vi "lapdata_new.vi"(6 "Reset":bool, 7 "Laptrigger":bool, 8 "InverterTemps":dbl[](array[numeric]), 9 "MotorTemps":dbl[](array[numeric]), 10 "Current":dbl, 11 "Hv Data":dbl[](array[numeric])) -> (0 "Inverter Temp":cluster{i32[], dbl[]}[](graph), 1 "Motor Temp":cluster{i32[], dbl[]}[](graph), 2 "HV Temps":dbl[](array[numeric]), 3 "Lap                    Laptime                        SoC                 Current Avg |                             Motor Temperatures                          |                               Inverter Temperatures":T1(array[cluster]) {"Laptime" format="%<%M:%S%2u>T"})   [LabVIEW 2017]
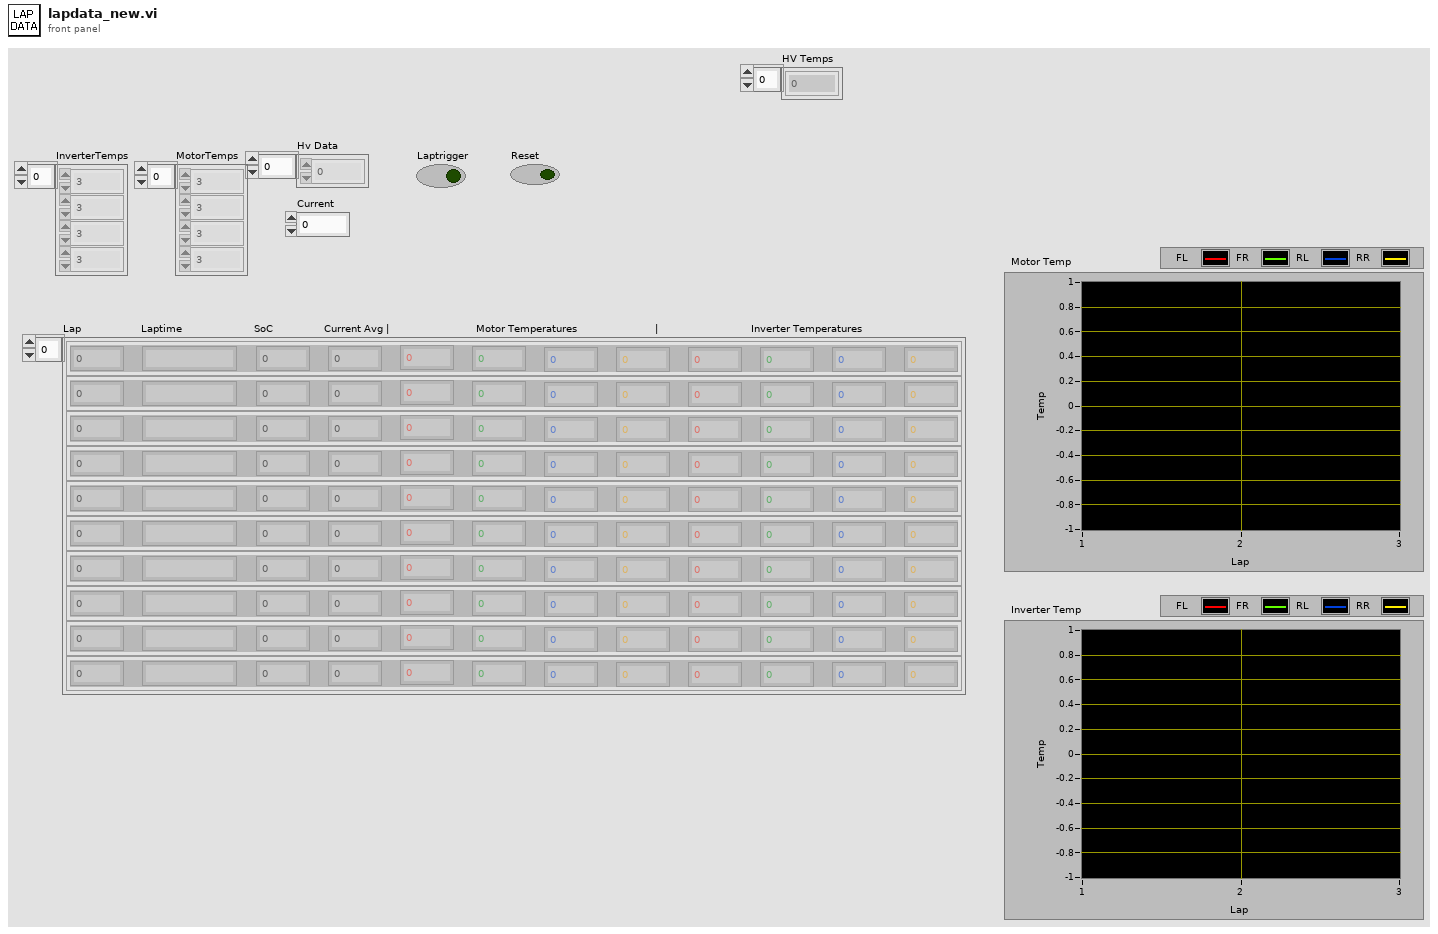
[diagram p1: front panel]
types:
  T1 = cluster{"SoC":i32, "MotorTemp_FL":dbl, "MotorTemp_FR":dbl, "MotorTemp_RL":dbl, "MotorTemp_RR":dbl, "InverterTemp_FL":dbl, "InverterTemp_FR":dbl, "InverterTemp_RL":dbl, "InverterTemp_RR":dbl, "Laptime":timestamp, "Lap":i32, "Curr Abs Avg":dbl}[]
  T2 = cluster{"SoC":i32, "MotorTemp_FL":dbl, "MotorTemp_FR":dbl, "MotorTemp_RL":dbl, "MotorTemp_RR":dbl, "InverterTemp_FL":dbl, "InverterTemp_FR":dbl, "InverterTemp_RL":dbl, "InverterTemp_RR":dbl, "Laptime":timestamp, "Lap":i32, "Current Abs Avg":dbl, "HV Temp":dbl}[]
  T3 = cluster{"SoC":i32, "MotorTemp_FL":dbl, "MotorTemp_FR":dbl, "MotorTemp_RL":dbl, "MotorTemp_RR":dbl, "InverterTemp_FL":dbl, "InverterTemp_FR":dbl, "InverterTemp_RL":dbl, "InverterTemp_RR":dbl, "Laptime":timestamp, "Lap":i32, "Current Abs Avg":dbl, "HV Temp":dbl}
  T4 = cluster{"SoC":i32, "MotorTemp_FL":dbl, "MotorTemp_FR":dbl, "MotorTemp_RL":dbl, "MotorTemp_RR":dbl, "InverterTemp_FL":dbl, "InverterTemp_FR":dbl, "InverterTemp_RL":dbl, "InverterTemp_RR":dbl, "Laptime":timestamp, "Lap":i32, "Current Abs Avg":dbl}
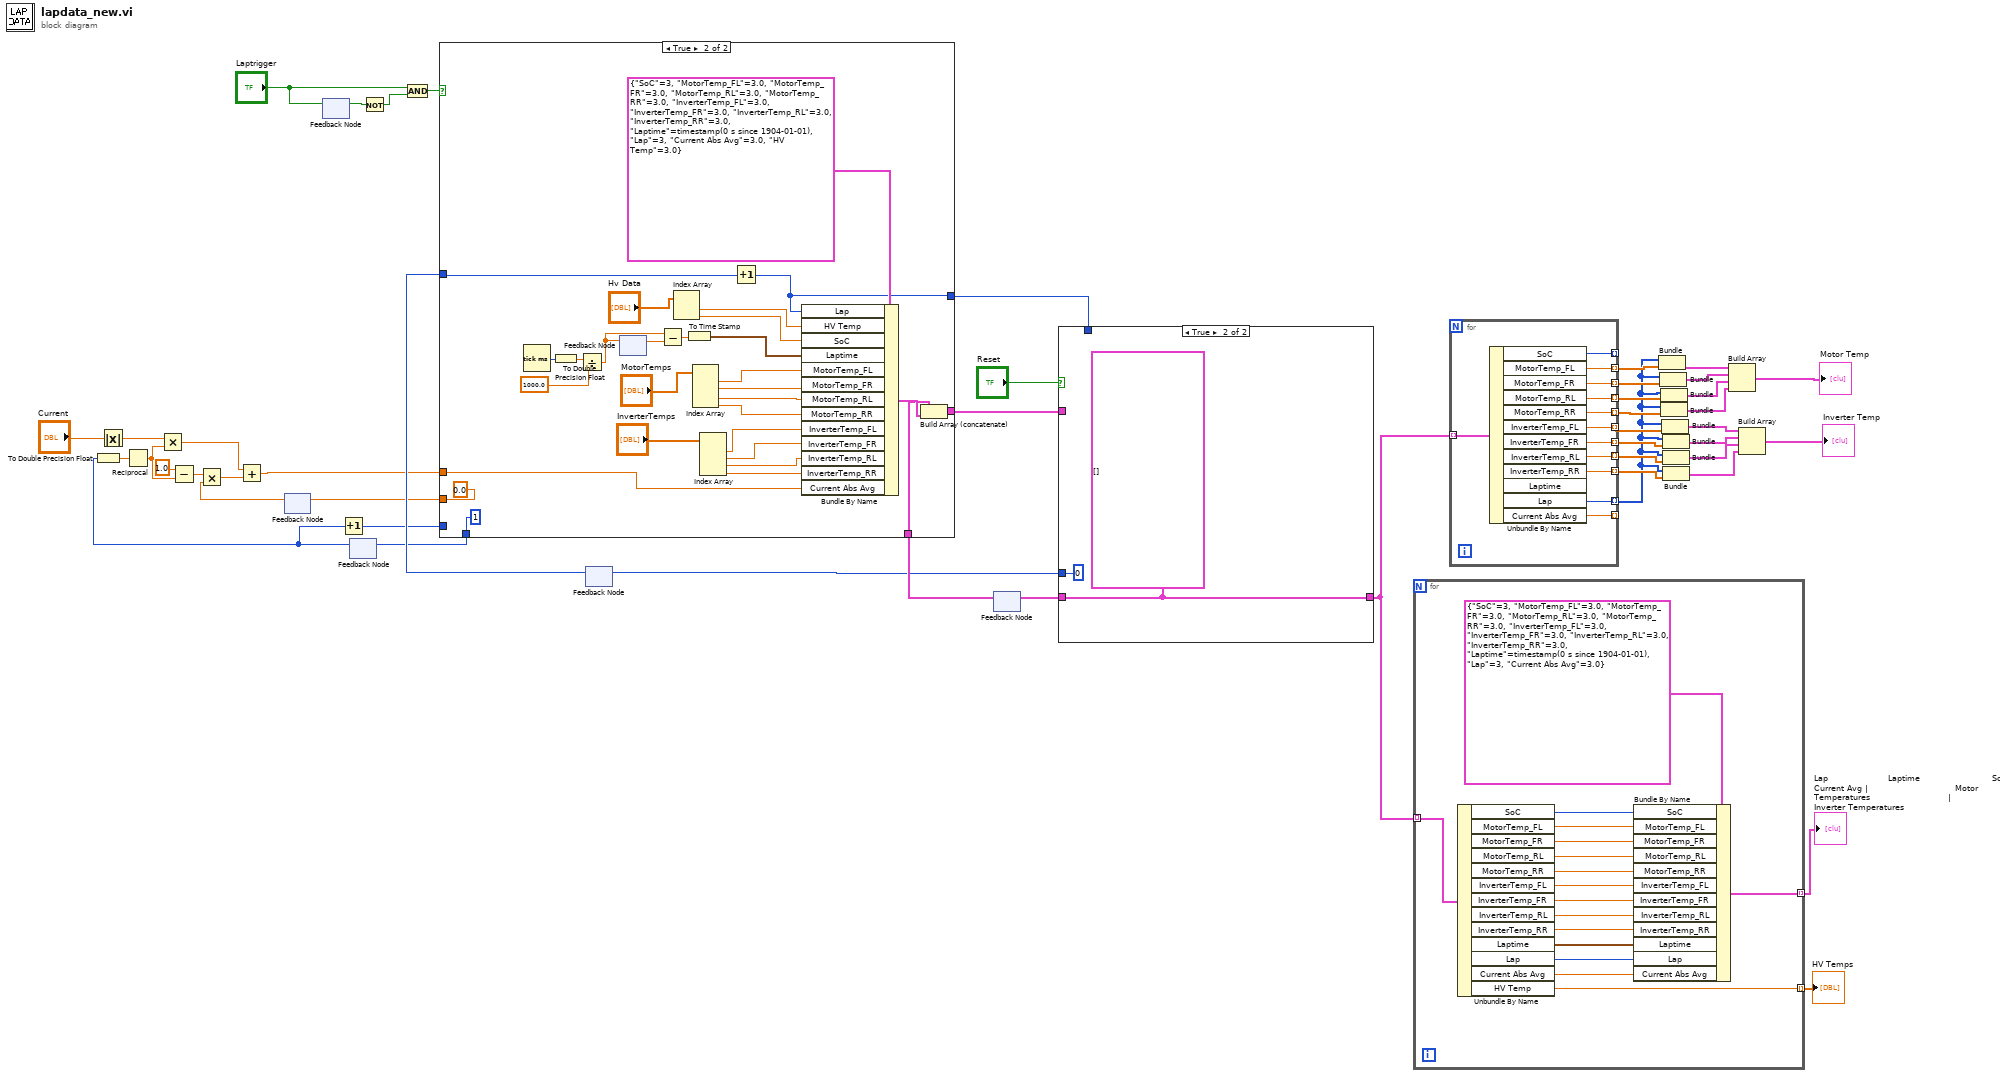
[diagram p0: block diagram]
diagram:
  n1 = Absolute Value(x="Current") -> (abs(x)=w28:dbl)
  n2 = feedback #1() -> (w32:dbl)  [unwired: 1 in]
  n3 = feedback #2() -> (w46:bool)  [unwired: 1 in]
  n4 = feedback-in #2("Laptrigger") -> ()
  n5 = feedback #3() -> (w35:i32)  [unwired: 1 in]
  n6 = To Double Precision Float(number=w35) -> (double precision float=w36:dbl)
  n7 = Reciprocal(x=w36) -> (1/x=w30:dbl)
  n8 = Multiply(x=w28, y=w30) -> (x*y=w34:dbl)
  n9 = Subtract(x=1.0, y=w30) -> (x-y=w31:dbl)
  n10 = Multiply(x=w31, y=w32) -> (x*y=w33:dbl)
  n11 = Add(x=w34, y=w33) -> (x+y=w24:dbl)
  n12 = Increment(x=w35) -> (x+1=w26:i32)
  n13 = Not(x=w46) -> (.not. x?=w45:bool)
  n14 = And(x="Laptrigger", y=w45) -> (x .and. y?=w43:bool)
  n15 = feedback #4() -> (w37:i32)  [unwired: 1 in]
  n16 = feedback #5() -> (w47:T2)  [unwired: 1 in]
  n17 = case shown="True" w43 {
    tunnel: w47 -> [w51 w60]
    tunnel: [w51 w79] -> w41
    tunnel: [w50 w53] -> w39
    tunnel: w37 -> [w50 w59]
    tunnel: w26 -> [w49 _]
    tunnel: [w49 1 ("Lap")] -> w25
    tunnel: w24 -> [w48 w56]
    tunnel: [w48 0.0] -> w23
    frame False {
    }
    frame True {
      n18 = Tick Count (ms)() -> (millisecond timer value=w68:u32)
      n19 = To Double Precision Float(number=w68) -> (double precision float=w67:dbl)
      n20 = Divide(x=w67, y=1000.0) -> (x/y=w64:dbl)
      n21 = feedback #6() -> (w65:dbl)  [unwired: 1 in]
      n22 = feedback-in #6(w64) -> ()
      n23 = Subtract(x=w64, y=w65) -> (x-y=w63:dbl)
      n24 = Index Array(array="Hv Data") -> (element #1=w52:dbl, element #2=w54:dbl)  [unwired: 2 in]
      n25 = To Time Stamp(1:w63) -> (0:w62:timestamp)
      n26 = Index Array(array="MotorTemps") -> (element #1=w77:dbl, element #2=w76:dbl, element #3=w75:dbl, element #4=w74:dbl)  [unwired: 4 in]
      n27 = Index Array(array="InverterTemps") -> (element #1=w72:dbl, element #2=w71:dbl, element #3=w70:dbl, element #4=w69:dbl)  [unwired: 4 in]
      n28 = Increment(x=w59) -> (x+1=w53:i32)
      n29 = Bundle By Name(cluster=T3 {"SoC"=3, "MotorTemp_FL"=3.0, "MotorTemp_FR"=3.0, "MotorTemp_RL"=3.0, "MotorTemp_RR"=3.0, "InverterTemp_FL"=3.0, "InverterTemp_FR"=3.0, "InverterTemp_RL"=3.0, "InverterTemp_RR"=3.0, "Laptime"=timestamp(0 s since 1904-01-01), "Lap"=3, "Current Abs Avg"=3.0, "HV Temp"=3.0}, "Lap"=w53, "HV Temp"=w52, "SoC"=w54, "Laptime"=w62, "MotorTemp_FL"=w77, "MotorTemp_FR"=w76, "MotorTemp_RL"=w75, "MotorTemp_RR"=w74, "InverterTemp_FL"=w72, "InverterTemp_FR"=w71, "InverterTemp_RL"=w70, "InverterTemp_RR"=w69, "Current Abs Avg"=w56) -> (w61:T3)
      n30 = Build Array (concatenate)(w60, w61) -> (w79:T2)
    }
  }
  n31 = feedback-in #1(w23) -> ()
  n32 = feedback-in #3(w25) -> ()
  n33 = case shown="True" "Reset" {
    tunnel: [w82 w83] -> w40
    tunnel: w41 -> [w82 _]
    tunnel: [w82 w83] -> w3
    tunnel: w39 -> [w81 _]
    tunnel: [w81 0 ("Lap")] -> w38
    frame False {
    }
    frame True {
      w83 = T2 []
    }
  }
  n34 = feedback-in #4(w38) -> ()
  n35 = feedback-in #5(w40) -> ()
  n36 = for {
    tunnel: w3 -> [w100] mode=indexing
    tunnel: [w86] -> w2 mode=indexing
    tunnel: [w85] -> w1 mode=indexing
    n37 = Unbundle By Name(w100) -> ("SoC"=w98:i32, "MotorTemp_FL"=w97:dbl, "MotorTemp_FR"=w96:dbl, "MotorTemp_RL"=w95:dbl, "MotorTemp_RR"=w94:dbl, "InverterTemp_FL"=w93:dbl, "InverterTemp_FR"=w92:dbl, "InverterTemp_RL"=w91:dbl, "InverterTemp_RR"=w90:dbl, "Laptime"=w89:timestamp, "Lap"=w88:i32, "Current Abs Avg"=w87:dbl, "HV Temp"=w85:dbl)
    n38 = Bundle By Name(cluster=T4 {"SoC"=3, "MotorTemp_FL"=3.0, "MotorTemp_FR"=3.0, "MotorTemp_RL"=3.0, "MotorTemp_RR"=3.0, "InverterTemp_FL"=3.0, "InverterTemp_FR"=3.0, "InverterTemp_RL"=3.0, "InverterTemp_RR"=3.0, "Laptime"=timestamp(0 s since 1904-01-01), "Lap"=3, "Current Abs Avg"=3.0}, "SoC"=w98, "MotorTemp_FL"=w97, "MotorTemp_FR"=w96, "MotorTemp_RL"=w95, "MotorTemp_RR"=w94, "InverterTemp_FL"=w93, "InverterTemp_FR"=w92, "InverterTemp_RL"=w91, "InverterTemp_RR"=w90, "Laptime"=w89, "Lap"=w88, "Current Abs Avg"=w87) -> (w86:T4)
  }
  "Lap                    Laptime                        SoC                 Current Avg |                             Motor Temperatures                          |                               Inverter Temperatures" <- w2
  "HV Temps" <- w1
  n39 = for {
    tunnel: w3 -> [w112] mode=indexing
    tunnel: [w111] -> _ mode=indexing
    tunnel: [w110] -> w22 mode=indexing
    tunnel: [w109] -> w19 mode=indexing
    tunnel: [w108] -> w18 mode=indexing
    tunnel: [w107] -> w17 mode=indexing
    tunnel: [w106] -> w13 mode=indexing
    tunnel: [w105] -> w12 mode=indexing
    tunnel: [w104] -> w11 mode=indexing
    tunnel: [w103] -> w10 mode=indexing
    tunnel: [w102] -> _ mode=indexing
    tunnel: [w101] -> w4 mode=indexing
    n40 = Unbundle By Name(w112) -> ("SoC"=w111:i32, "MotorTemp_FL"=w110:dbl, "MotorTemp_FR"=w109:dbl, "MotorTemp_RL"=w108:dbl, "MotorTemp_RR"=w107:dbl, "InverterTemp_FL"=w106:dbl, "InverterTemp_FR"=w105:dbl, "InverterTemp_RL"=w104:dbl, "InverterTemp_RR"=w103:dbl, "Lap"=w101:i32, "Current Abs Avg"=w102:dbl)  [unwired: 1 out]
  }
  n41 = Bundle(w4, w22) -> (w21:cluster{i32[], dbl[]})  [unwired: 1 in]
  n42 = Bundle(w4, w19) -> (w16:cluster{i32[], dbl[]})  [unwired: 1 in]
  n43 = Bundle(w4, w18) -> (w15:cluster{i32[], dbl[]})  [unwired: 1 in]
  n44 = Bundle(w4, w17) -> (w14:cluster{i32[], dbl[]})  [unwired: 1 in]
  n45 = Bundle(w4, w13) -> (w8:cluster{i32[], dbl[]})  [unwired: 1 in]
  n46 = Bundle(w4, w12) -> (w7:cluster{i32[], dbl[]})  [unwired: 1 in]
  n47 = Bundle(w4, w11) -> (w6:cluster{i32[], dbl[]})  [unwired: 1 in]
  n48 = Bundle(w4, w10) -> (w5:cluster{i32[], dbl[]})  [unwired: 1 in]
  n49 = Build Array(w21, w16, w15, w14) -> (→"Motor Temp":cluster{i32[], dbl[]}[])
  n50 = Build Array(w8, w7, w6, w5) -> (→"Inverter Temp":cluster{i32[], dbl[]}[])
